vi "Prefix error msg.vi"(7 "PrefixMessage":string, 10 "ErrorIn":errorcluster) -> (2 "ErrorOut":errorcluster)   [LabVIEW 2021, in "YActor.lvclass"]
uses:
  YActor.lvclass
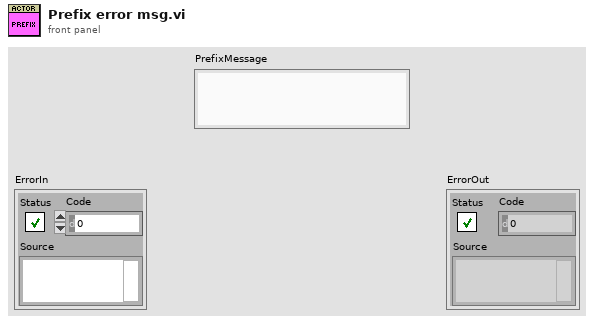
[diagram p1: front panel]
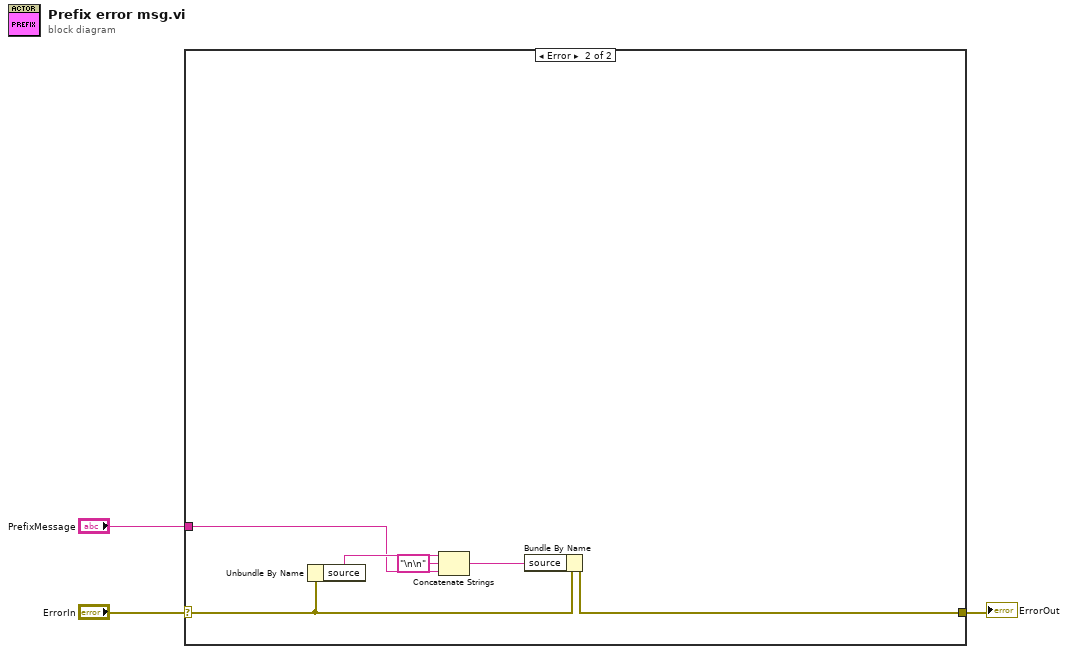
[diagram p0: block diagram]
diagram:
  n1 = case shown="Error" "ErrorIn" {
    selector: "ErrorIn" -> [w4 w10]
    tunnel: [w4 w9] -> w2
    tunnel: "PrefixMessage" -> [_ w5]
    frame No Error {
    }
    frame Error {
      n2 = Unbundle By Name(w10) -> ("source"=w6:string)
      n3 = Concatenate Strings(w6, "\n\n" ("string"), w5) -> (w7:string)
      n4 = Bundle By Name(cluster=w10, "source"=w7) -> (w9:errorcluster)
    }
  }
  "ErrorOut" <- w2
